vi "Handle SearchPage Mouse Move.vi"(0 "Vertical Coordinate":i32, 1 "Horizontal Coordinate":i32, 3 "List Item Height":i16, 4 "Row with Hover Link in":i32, 6 "Scrollbar Refnum":refnum<vi>, 7 "Desc Link Character Index Array":i32[](array[numeric]), 8 "Draw Area Size":T1, 10 "Project List Refnum":refnum<vi>, 11 "Searched Templates":refnum<class "MetaDataObj.lvclass">[](array[class]), 12 "Main VI Refnum":refnum<vi>, 13 "Index into All T's":i32[](array[numeric])) -> (14 "Messages":string[](array[string]), 18 "Row with Hover Link out":i32)   [LabVIEW 2016]
uses:
  <resource>/dialog/NewProjectWizard/MetaDataObj/MetaDataObj.lvclass
  <vilib>/Utility/miscctls.llb/LVBoundsTypeDef.ctl
  <vilib>/Utility/cursorutil.llb/Set Cursor (Icon Pict).vi
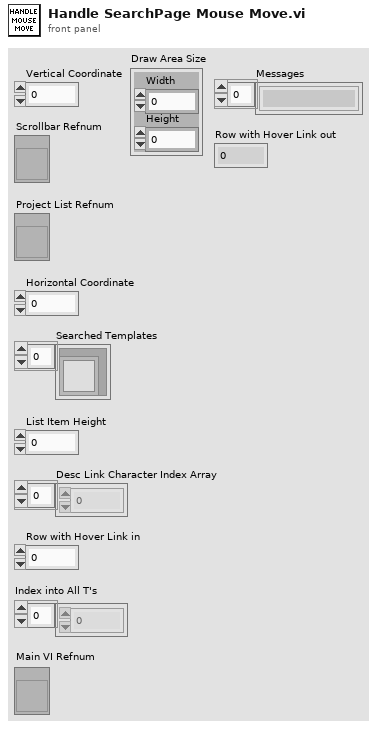
[diagram p1: front panel]
types:
  T1 = typedef "LVBoundsTypeDef.ctl" = cluster{"Width":u32, "Height":u32}
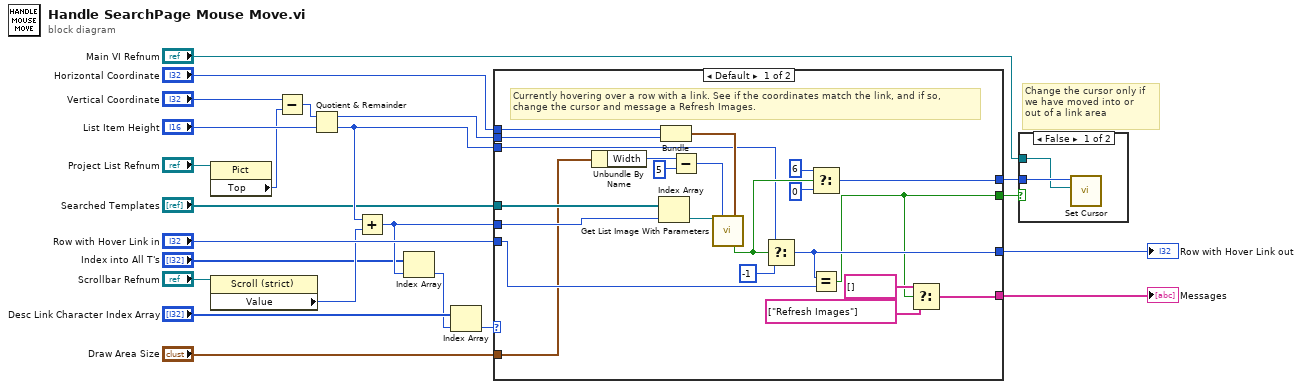
[diagram p0: block diagram]
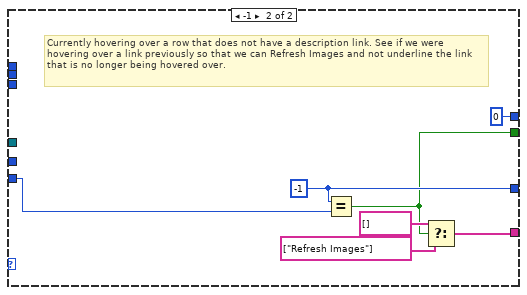
[diagram p3: hidden frame]
diagram:
  # "Change the cursor only if\nwe have moved into or\nout of a link area"
  n1 = property on="Property Node" class="Pict"(reference="Project List Refnum") -> ("Top"=w9:i32)  [unwired: 1 in, 2 out]
  n2 = property class="Scroll (strict)"(reference="Scrollbar Refnum") -> ("Value"=w8:i32)  [unwired: 1 in, 2 out]
  n3 = Subtract(x="Vertical Coordinate", y=w9) -> (x-y=w10:i32)
  n4 = Quotient & Remainder(x=w10, y="List Item Height") -> (x-y*floor(x/y)=w17:i32, floor(x/y)=w23:i32)
  n5 = Add(x=w23, y=w8) -> (x+y=w4:i32)
  n6 = Index Array(array="Index into All T's", index=w4) -> (element=w2:i32)
  n7 = Index Array(array="Desc Link Character Index Array", index=w2) -> (element=w13:i32)
  n8 = case shown="Default" w13 {
    tunnel: "Searched Templates" -> [w45 _]
    tunnel: "Horizontal Coordinate" -> [w38 _]
    tunnel: w17 -> [w39 _]
    tunnel: w4 -> [w29 _]
    tunnel: [w35 u16 0] -> w22
    tunnel: [w27 w51] -> w18
    tunnel: "Row with Hover Link in" -> [w33 w50]
    tunnel: [w30 w47] -> w20
    tunnel: [w26 w46] -> w21
    tunnel: w23 -> [w25 _]
    tunnel: "Draw Area Size" -> [w24 _]
    frame Default {
      # "Currently hovering over a row with a link. See if the coordinates match the link, and if so,\nchange the cursor and message a Refresh Images."
      n9 = Unbundle By Name(w24) -> ("Width"=w41:u32)
      n10 = Index Array(array=w45, index=w29) -> (element=w43:refnum<class "MetaDataObj.lvclass">)
      n11 = Bundle("Horizontal Coordinate"=w38, w39) -> (w44:cluster{"Horizontal Coordinate":i32, i32})  [unwired: 1 in]
      n12 = Subtract(x=w41, y=u32 5) -> (x-y=w40:u32)
      n13 = call <resource>:"Get List Image With Parameters.vi"("Template in"=w43, "Img Width"=w40, "DNL_Point"=w44) -> ("Hovering Over Link?"=w34:bool)  [unwired: 8 in, 4 out]
      n14 = Select(t=w25, s=w34, f=-1) -> (s? t:f=w27:i32)
      n15 = Select(t=u16 6, s=w34, f=u16 0) -> (s? t:f=w35:u16)
      n16 = Equal?(x=w27, y=w33) -> (x = y?=w26:bool)
      n17 = Select(t=string[] [], s=w26, f=string[] ["Refresh Images"]) -> (s? t:f=w30:string[])
    }
    frame -1 {
      w51 = -1
      # "Currently hovering over a row that does not have a description link. See if we were hovering over a link previously so that we can Refresh Images and not underline the link that is no longer being hovered over."
      n18 = Equal?(x=w51, y=w50) -> (x = y?=w46:bool)
      n19 = Select(t=string[] [], s=w46, f=string[] ["Refresh Images"]) -> (s? t:f=w47:string[])
    }
  }
  "Messages" <- w20
  "Row with Hover Link out" <- w18
  n20 = case shown="False" w21 {
    tunnel: w22 -> [w54 _]
    tunnel: "Main VI Refnum" -> [w53 _]
    frame False {
      n21 = call-poly <vilib>:"Set Cursor.vi"("VI reference (current VI)"=w53, "icon"=w54) -> ()  [unwired: 8 in, 2 out]
    }
    frame True {
    }
  }
